vi "Project1HandIn.vi"() -> ()   [LabVIEW 2024]
panel:
  out "AtoD":i16 format="%04x"
  in  "stop":bool
  out "GOOD":bool
  out "LOW":bool
  out "HIGH":bool
  out "Relative Humidity, %":dbl(slide) scale=0.0..100.0 scale format="%#_5f"
  out "Rsens, kOhm":dbl(slide) scale=20.0..40.0
  out "V+, V":dbl(slide) scale=2.0..3.5 scale format="%#_3f"
  out "vDiff,V":dbl(slide) scale=-0.1..0.5 scale format="%1.1f"
  out "Vscc":dbl(slide) scale=-7.5..7.5 scale format="%1.3f"
  # "Technical items"
  # "User interface"
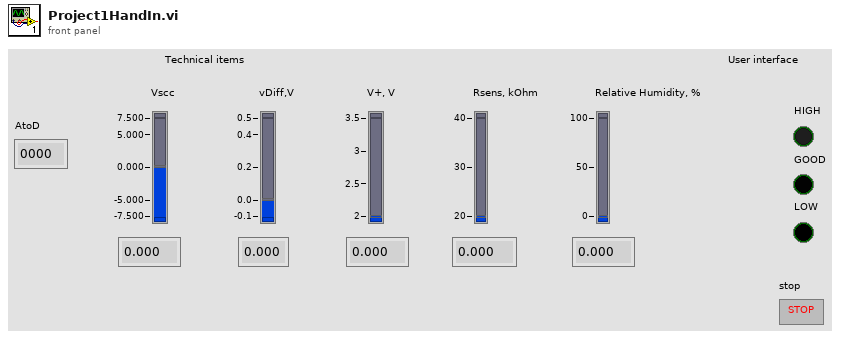
[diagram p1: front panel]
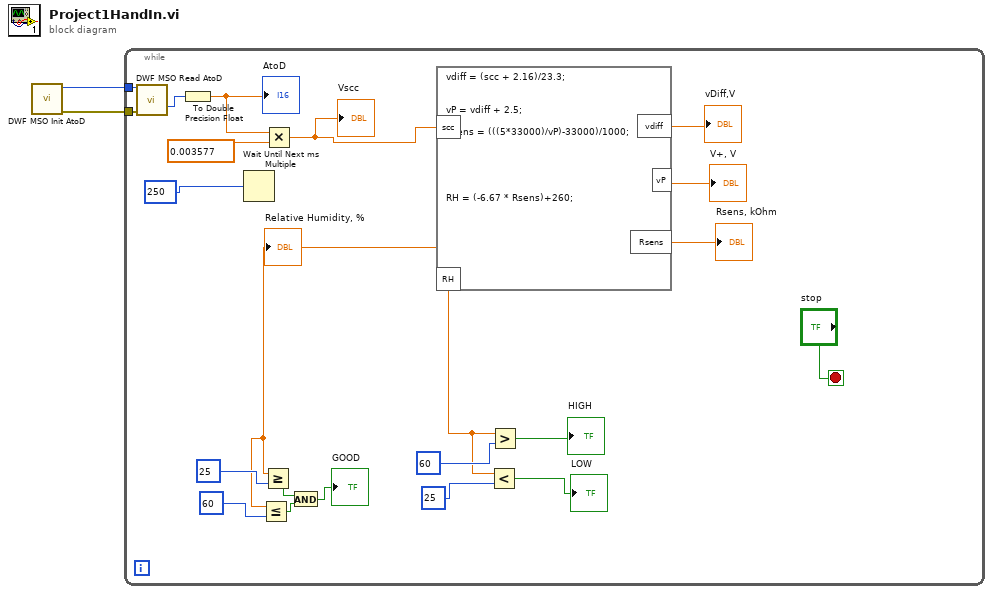
[diagram p0: block diagram]
diagram:
  n1 = call "DWF MSO Init AtoD.vi"() -> ("Error Out"=w1:errorcluster, "Instrument Handle Out"=w2:u32)  [unwired: 10 in]
  n2 = while {
    tunnel: w2 -> [w5]
    tunnel: w1 -> [w4]
    stop <- "stop" stop-if-true
    n3 = call "DWF MSO Read AtoD.vi"("Instrument Handle In AtoD"=w5, "Error In"=w4) -> ("AtoD"=w6:i16)  [unwired: 12 in, 1 out]
    n4 = To Double Precision Float(number=w6) -> (double precision float=w22:dbl)
    "AtoD" <- w22
    n5 = Wait Until Next ms Multiple(millisecond multiple=250) -> ()  [unwired: 1 out]
    n6 = Multiply(x=w22, y=0.003577) -> (x*y=w20:dbl)
    "Vscc" <- w20
    n7 = formula code="vdiff = (scc + 2.16)/23.3;\n\n\nvP = vdiff + 2.5;\n\nRsens = (((5*33000)/vP)-33000)/1000;\n\n\n\n\n\nRH = (-6.67 * Rsens)+260;"("scc"=w20) -> ("vdiff"=→"vDiff,V":dbl, "vP"=→"V+, V":dbl, "Rsens"=→"Rsens, kOhm":dbl, "RH"=w11:dbl)
    "Relative Humidity, %" <- w11
    n8 = Less Or Equal?(x=w11, y=60) -> (x <= y?=w9:bool)
    n9 = Greater Or Equal?(x=w11, y=25) -> (x >= y?=w8:bool)
    n10 = And(x=w8, y=w9) -> (x .and. y?=→"GOOD":bool)
    n11 = Less?(x=w11, y=25) -> (x < y?=→"LOW":bool)
    n12 = Greater?(x=w11, y=60) -> (0:→"HIGH":bool)
  }
